vi "Get Value and Valid.vi"(8 "error in (no error)":errorcluster, 11 "Dynamic Combobox in":refnum<class "Dynamic Combobox.lvclass">) -> (0 "error out":errorcluster, 1 "Valid":bool, 2 "Value":string, 3 "Dynamic Combobox out":refnum<class "Dynamic Combobox.lvclass">)   [LabVIEW 2020, in "Dynamic Combobox.lvlib" / "Dynamic Combobox.lvclass"]
uses:
  Dynamic Combobox.lvclass
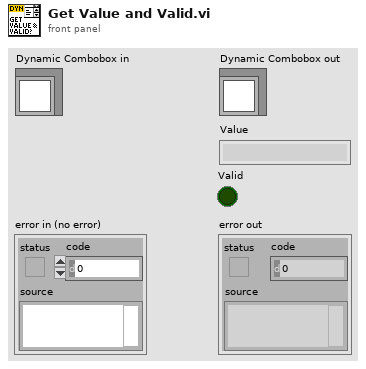
[diagram p1: front panel]
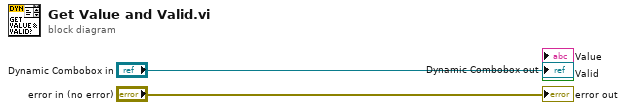
[diagram p0: block diagram]
diagram:
  "error out" <- "error in (no error)"
  "Dynamic Combobox out" <- "Dynamic Combobox in"
